vi "Close.vi"(8 "error in (no error)":errorcluster, 11 "PROFIBUS in":refnum<class "Profibus.lvclass">) -> (0 "error out":errorcluster, 3 "PROFIBUS out":refnum<class "Profibus.lvclass">)   [LabVIEW 2016, in "Profibus.lvclass"]
uses:
  Profibus.lvclass
  Profibus VISA Driver/DF PROFI II.llb/DFP2_Initialisation.ctl
  Profibus.lvclass/Profibus.ctl
  Protocol Class/Protocol.lvclass
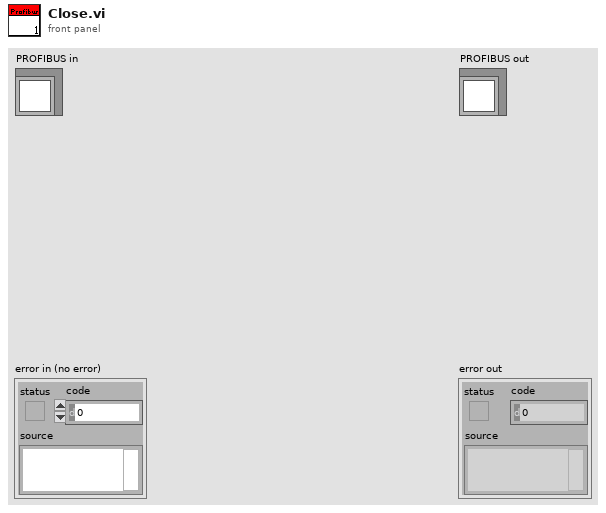
[diagram p1: front panel]
types:
  T1 = typedef "DFP2_Initialisation.ctl" = enum32{"InitDFProfiIIAsDP-Master", "InitDFProfiIIAsDP-Slave", "Abort"}
  T2 = cluster{"Error":bool, "Status":i32, "Info":string}
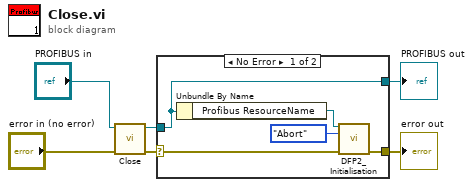
[diagram p0: block diagram]
diagram:
  n1 = call-parent "Close.vi"("error in (no error)"="error in (no error)", "Protocol in"="PROFIBUS in") -> ("error out"=w4:errorcluster, "Protocol out"=w2:refnum<class "Profibus.lvclass">)  [unwired: 8 in]
  n2 = case shown="No Error" w4 {
    selector: w4 -> [w7 w13]
    tunnel: [w9 w13] -> w3
    tunnel: w2 -> [w11 w12]
    tunnel: [w11 w12] -> w1
    frame No Error {
      n3 = Unbundle By Name(w11) -> ("Profibus ResourceName"=w8:refnum<visa-resource-name>)
      n4 = call "DFP2_Initialisation.vi"("DFP2ResourceName"=w8, "Mode"=DFP2_Initialisation."Abort", "ErrorIn:"=w7) -> ("ErrorOut:"=w9:T2)  [unwired: 10 in, 2 out]
    }
    frame Error {
    }
  }
  "error out" <- w3
  "PROFIBUS out" <- w1
